vi "AddQ.vi"(8 "error in (no error)":errorcluster, 10 "QNames":string[](array[string])) -> (0 "error out":errorcluster, 2 "dCVT QMH out":T1)   [LabVIEW 2020, in "QDict.lvlib"]
doc: "Developed by Kevin Thompson\nkevin@thompsonengineering.net\n\nCopyright 2021\nThompson Engineering, LLC"
uses:
  QDict.lvlib
  <vilib>/TELLC/Dynamic CVT API/TD Dynamic CVT DVR--ref.ctl
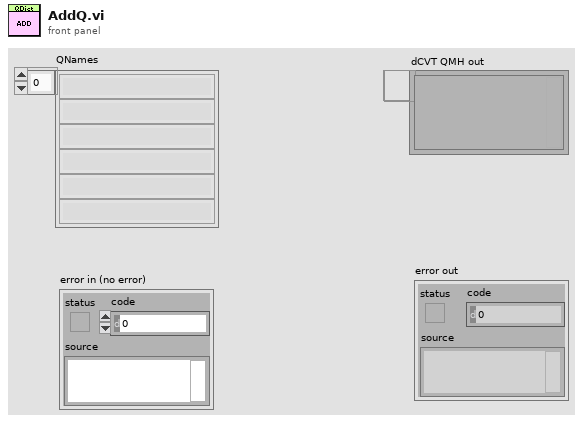
[diagram p1: front panel]
types:
  T1 = typedef "TD Dynamic CVT DVR--ref.ctl" = refnum<data-value>
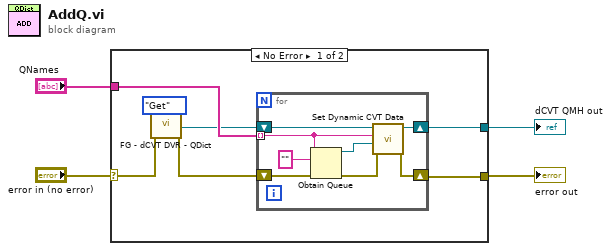
[diagram p0: block diagram]
diagram:
  n1 = case shown="No Error" "error in (no error)" {
    selector: "error in (no error)" -> [w7 w21]
    tunnel: "QNames" -> [w11 _]
    tunnel: [w5 T1 refnum ("dCVT QMsg out")] -> w3
    tunnel: [w6 w21] -> w2
    frame No Error {
      n2 = call "FG - dCVT DVR - QDict.vi"("error in (no error)"=w7, "Action (Get)"=enum16{"Init", "Get", "Set"}."Get") -> ("dCVT QMH out"=w9:T1, "error out"=w8:errorcluster)  [unwired: 7 in]
      n3 = for {
        tunnel: w11 -> [w16] mode=indexing
        shift-right: [w14] -> w6
        shift-left: w8 -> [w18]
        shift-right: [w13] -> w5
        shift-left: w9 -> [w12]
        n4 = Obtain Queue(name (unnamed)=w16, element data type="", error in (no error)=w18) -> (queue out=w15:refnum<queue>, error out=w17:errorcluster)  [unwired: 2 in, 1 out]
        n5 = call <vilib>:"Set Dynamic CVT Data.vi"("error in (no error)"=w17, "value"=w15, "DataName"=w16, "dCVT DVR"=w12) -> ("error out"=w14:errorcluster, "dCVT DVR out"=w13:T1)  [unwired: 5 in, 1 out]
      }
    }
    frame Error {
    }
  }
  "dCVT QMH out" <- w3
  "error out" <- w2
